vi "checkMCodeConfig.vi"(11 "INPUT":string) -> (1 "MCODE":dbl, 3 "OUTPUT":string)   [LabVIEW 2017]
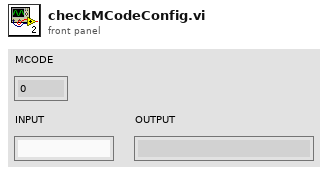
[diagram p1: front panel]
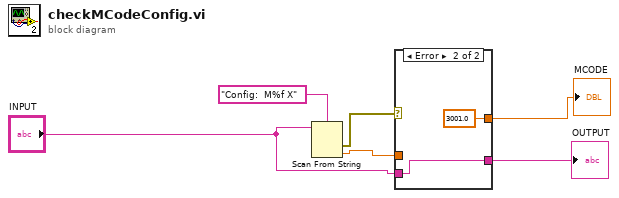
[diagram p0: block diagram]
diagram:
  n1 = Scan From String(format string="Config:  M%f X", input string="INPUT") -> (error out=w3:errorcluster, output 1=w1:dbl)  [unwired: 3 in, 2 out]
  n2 = case shown="Error" w3 {
    tunnel: "INPUT" -> [w8 w9]
    tunnel: [w8 w9] -> w4
    tunnel: [w7 3001.0] -> w2
    tunnel: w1 -> [w7 _]
    frame No Error {
    }
    frame Error {
    }
  }
  "OUTPUT" <- w4
  "MCODE" <- w2
